vi "WPI_RobotDriveOpen2Motor.vi"   [LabVIEW 2017]
doc: "Opens a reference to the robot drive for a two-motor robot using Talon, Victor, Jaguar, or \"Exisiting\" motor controllers. Robot Drive Open configures both motors (with the exception of <B>Existing Motors</B>). You must open a reference before using any other VIs on this palette.\n\nThis software is licensed. Open the labview\\readme\\WPI Robotics Library Open Source License.txt file for more information."
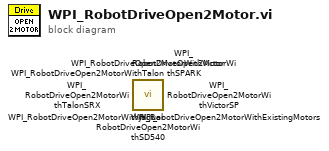
[diagram p0: block diagram]
diagram:
  n1 = call <vilib>:"WPI_RobotDriveOpen2MotorWithSD540.vi"() -> ()  [unwired: 10 in, 2 out]
  n2 = call <vilib>:"WPI_RobotDriveOpen2MotorWithSPARK.vi"() -> ()  [unwired: 10 in, 2 out]
  n3 = call <vilib>:"WPI_RobotDriveOpen2MotorWithTalonSRX.vi"() -> ()  [unwired: 10 in, 2 out]
  n4 = call <vilib>:"WPI_RobotDriveOpen2MotorWithVictorSP.vi"() -> ()  [unwired: 10 in, 2 out]
  n5 = call <vilib>:"WPI_RobotDriveOpen2MotorWithTalon.vi"() -> ()  [unwired: 10 in, 2 out]
  n6 = call <vilib>:"WPI_RobotDriveOpen2MotorWithExistingMotors.vi"() -> ()  [unwired: 10 in, 2 out]
  n7 = call <vilib>:"WPI_RobotDriveOpen2MotorWithVictor.vi"() -> ()  [unwired: 10 in, 2 out]
  n8 = call <vilib>:"WPI_RobotDriveOpen2MotorWithJaguar.vi"() -> ()  [unwired: 10 in, 2 out]
